vi "mqttUserInfoWrite.vi"(0 "mqtt in":refnum<class "mqtt.lvclass">, 5 "User Info":T1={"User Name"="User", "Password"="password"}, 11 "error in (no error)":errorcluster) -> (4 "mqtt out":refnum<class "mqtt.lvclass">, 15 "error out":errorcluster)   [LabVIEW 2018, in "mqtt.lvclass"]
uses:
  mqtt.lvclass
  mqttTypedef/mqttWillInformation.ctl
  mqtt.lvclass/mqtt.ctl
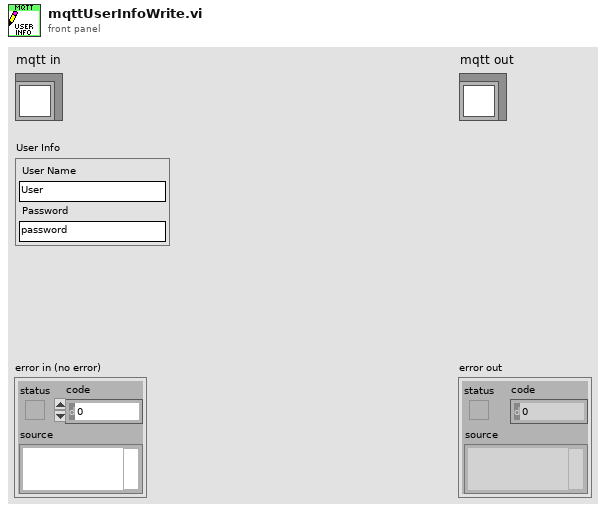
[diagram p1: front panel]
types:
  T1 = typedef "mqttWillInformation.ctl" = cluster{"User Name":string, "Password":string}
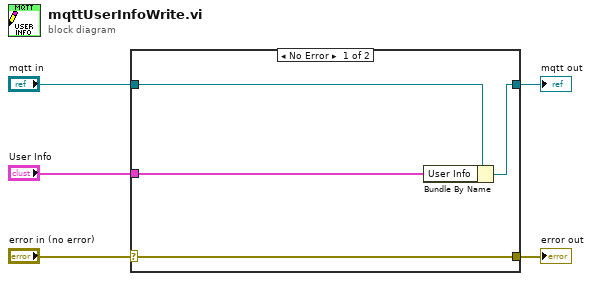
[diagram p0: block diagram]
diagram:
  n1 = case shown="No Error" "error in (no error)" {
    selector: "error in (no error)" -> [w9 w10]
    tunnel: [w9 w10] -> w4
    tunnel: [w7 w11] -> w2
    tunnel: "mqtt in" -> [w8 w11]
    tunnel: "User Info" -> [w6 _]
    frame No Error {
      n2 = Bundle By Name(cluster=w8, "User Info"=w6) -> (w7:refnum<class "mqtt.lvclass">)
    }
    frame Error {
    }
  }
  "error out" <- w4
  "mqtt out" <- w2
